vi "GFITS_Parse_2DARR.vi"(7 "Database RefNum in":T1, 11 "array in":string[][](table)) -> (3 "array out":string[][](table))   [LabVIEW 2016]
uses:
  DBSHAND/private/vis/DatabaseHand_RefNum.ctl
  DBSHAND/private/vis/DatabaseHand_Element_Get(string).vi
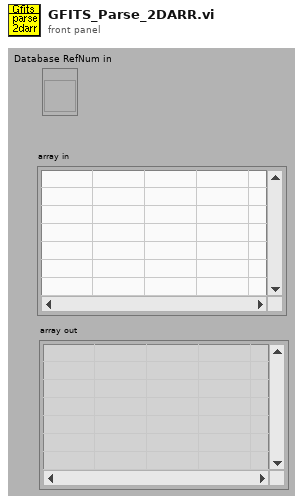
[diagram p1: front panel]
types:
  T1 = typedef "DatabaseHand_RefNum.ctl" = refnum<vi>
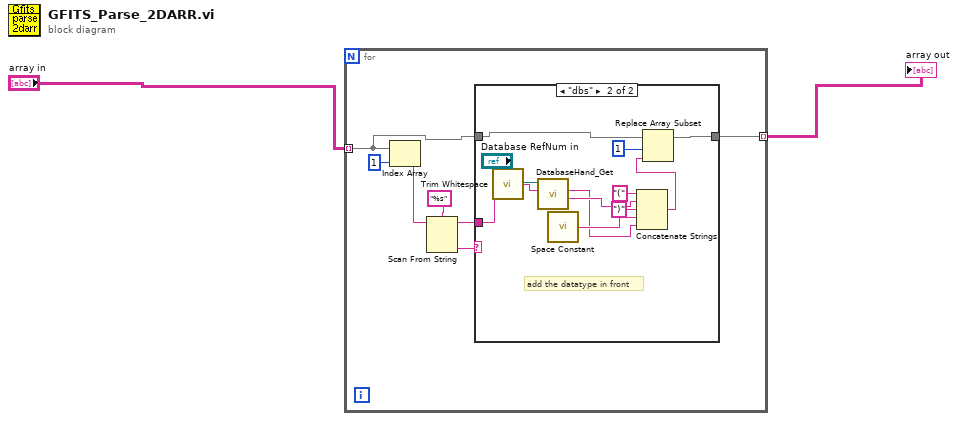
[diagram p0: block diagram]
diagram:
  n1 = for {
    tunnel: "array in" -> [w3] mode=indexing
    tunnel: [w5] -> w1 mode=indexing
    n2 = Index Array(array=w3, index=1) -> (element=w6:string)
    n3 = Scan From String(format string="%s", input string=w6) -> (remaining string=w4:string, output 1=w7:string)  [unwired: 2 in, 3 out]
    n4 = case shown="\"dbs\"" w7 {
      tunnel: w3 -> [w10 w11]
      tunnel: [w10 w18] -> w5
      tunnel: w4 -> [_ w21]
      frame Default {
      }
      frame "dbs" {
        # "add the datatype in front"
        n5 = call <vilib>:"Trim Whitespace.vi"("string"=w21) -> ("trimmed string"=w20:string)  [unwired: 1 in]
        n6 = call-poly "DatabaseHand_Get.vi"("name"=w20, "Database RefNum in"="Database RefNum in") -> ("type"=w16:string, "value"=w13:string)  [unwired: 3 in, 5 out]
        n7 = call <vilib>:"Space Constant.vi"() -> ("String"=w14:string)
        n8 = Concatenate Strings("(" ("string"), w16, ")" ("string"), w14, w13) -> (w12:string)
        n9 = Replace Array Subset(array=w11, new element=w12, index=1) -> (w18:string[])
      }
    }
  }
  "array out" <- w1
